vi "init_motorsystem.vi"(7 "dimension names":string[](array[string]), 8 "error in (no error)":errorcluster caption="错误输入（无错误）", 9 "CAN node IDs":u32[](array[numeric]), 10 "device index":u32, 11 "MotorSystem 输入":refnum<class "MotorSystem.lvclass">) -> (0 "error out":errorcluster caption="错误输出", 3 "MotorSystem 输出":refnum<class "MotorSystem.lvclass">)   [LabVIEW 2016, in "MotionControl.lvlib" / "MotorSystem.lvclass"]
uses:
  <userlib>/MotionControl/MotorSystem/MotorSystem.lvclass
  <userlib>/MotionControl/MotorSystem/MotorSystem.lvclass/MotorSystem.ctl
  <userlib>/MotionControl/OneMotion/OneMotion.lvclass
  <userlib>/MotionControl/MotorSystem/MotionCluster.ctl
  <vilib>/Utility/config.llb/NI_LVConfig.lvlib
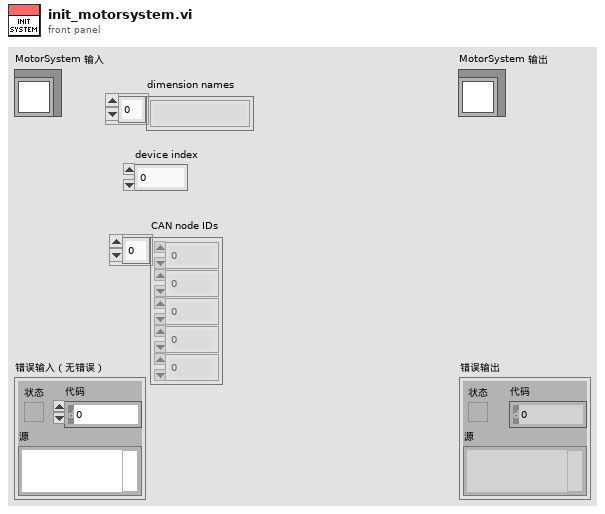
[diagram p1: front panel]
types:
  T1 = typedef "MotionControl.lvlib/MotorSystem.lvclass/MotionCluster.ctl" = cluster{"OneMotion.lvclass":refnum<class "OneMotion.lvclass">, "connected?":bool, "default enabled?":bool, "enabled?":bool}
  T2 = typedef "NI_LVConfig.lvlib/Config Data RefNum.ctl" = refnum<k1>
  T3 = typedef "MotionControl.lvlib/MotorSystem.lvclass/SavedPosCluster.ctl" = cluster{"name":string, "command list":T4}
  T4 = typedef "MotionControl.lvlib/MotorSystem.lvclass/CommandList.ctl" = cluster{"cmd":T5, "cmd info":T6[]}[]
  T5 = typedef "MotionControl.lvlib/MotorSystem.lvclass/cmd_system.ctl" = enum16{"NONE", "MOVE_SYSTEM", "WAIT_UNTIL_MOVE_DONE", "EXIT"}
  T6 = typedef "MotionControl.lvlib/MotorSystem.lvclass/SavedDimensionCluster.ctl" = cluster{"dimension name":string, "pos":dbl, "unit mode":T7, "unit conversion ratio":dbl}
  T7 = typedef "MotionControl.lvlib/OneMotion.lvclass/unit mode.ctl" = enum16{"motor (pulse)", "linear (mm) or radial (degree)"}
  T8 = cluster{"array for a soft limit":cluster{"dim name":string, "soft limit":cluster{"min":dbl, "max":dbl}}[]}[]
  T9 = cluster{"complete dimension names[0]":string, "complete dimension names[1]":string}
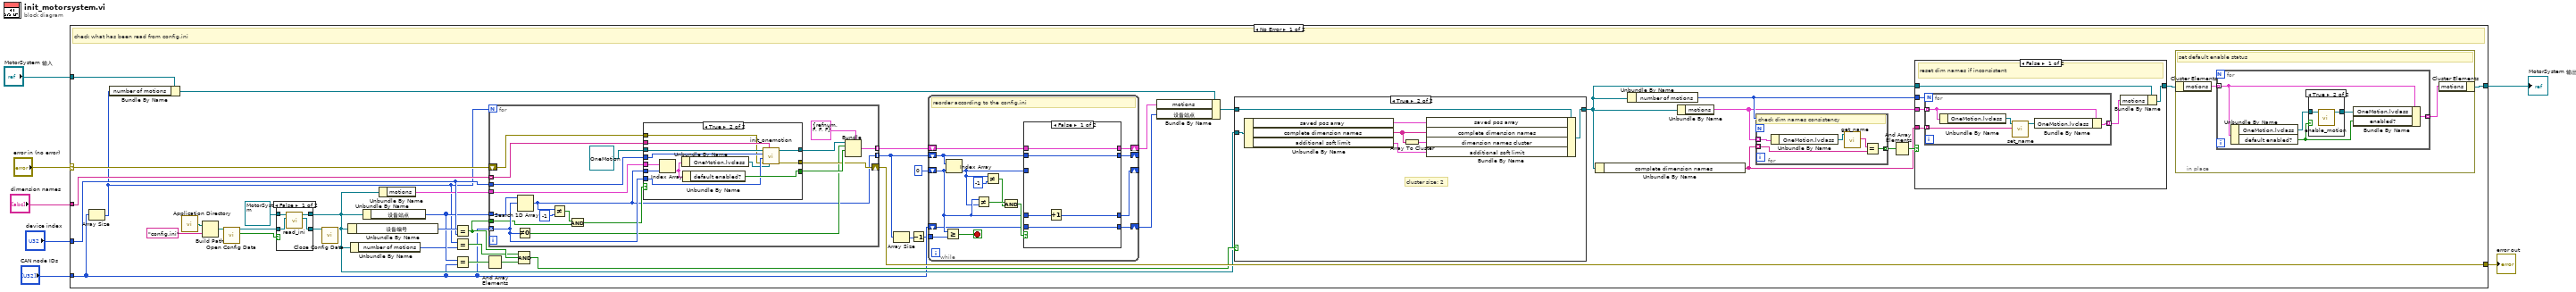
[diagram p0: block diagram]
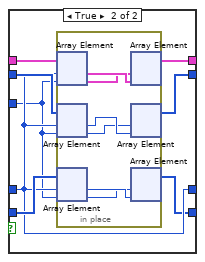
[diagram p2: hidden frame]
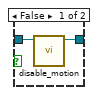
[diagram p3: hidden frame]
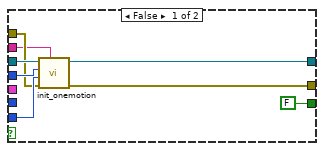
[diagram p7: hidden frame]
diagram:
  n1 = case shown="No Error" "error in (no error)" {
    selector: "error in (no error)" -> [w47 w164]
    tunnel: [w45 w164] -> w6
    tunnel: [w16 w163] -> w4
    tunnel: "MotorSystem 输入" -> [w46 w163]
    tunnel: "CAN node IDs" -> [w11 _]
    tunnel: "device index" -> [w36 _]
    tunnel: "dimension names" -> [w44 _]
    frame No Error {
      # "check what has been read from config.ini"
      n2 = Array Size(array=w11) -> (size(s)=w32:i32)
      n3 = Bundle By Name(cluster=w46, "number of motions"=w32) -> (w48:refnum<class "MotorSystem.lvclass">)
      n4 = call <vilib>:"Application Directory.vi"() -> ("Application Directory"=w43:path)
      n5 = Build Path(base path=w43, name or relative path="config.ini" ("名称或相对路径")) -> (appended path=w38:path)
      n6 = call <vilib>:"Open Config Data.vi"("configuration file path"=w38) -> ("file created?"=w18:bool, "refnum"=w41:T2)  [unwired: 8 in, 1 out]
      n7 = case shown="False" w18 {
        tunnel: w41 -> [w97 w98]
        tunnel: [w96 w98] -> w40
        tunnel: refnum<class "MotorSystem.lvclass"> refnum ("MotorSystem.lvclass") -> [w95 w99]
        tunnel: [w94 w99] -> w26
        frame False {
          n8 = call-dynamic "read_ini.vi"("file ref in"=w97, "MotorSystem 输入"=w95) -> ("file ref out"=w96:T2, "MotorSystem 输出"=w94:refnum<class "MotorSystem.lvclass">)  [unwired: 7 in, 1 out]
        }
        frame True {
        }
      }
      n9 = call <vilib>:"Close Config Data.vi"("refnum"=w40) -> ()  [unwired: 9 in, 2 out]
      n10 = Unbundle By Name(w26) -> ("设备编号"=w37:u32)
      n11 = Unbundle By Name(w26) -> ("number of motions"=w31:i32)
      n12 = Unbundle By Name(w26) -> ("设备站点"=w34:u32[])
      n13 = Unbundle By Name(w26) -> ("motions"=w35:T1[])
      n14 = Equal?(x=w37, y=w36) -> (x = y?=w30:bool)
      n15 = Equal?(x=w32, y=w31) -> (x = y?=w29:bool)
      n16 = Equal?(x=w34, y=w11) -> (x = y?=w33:bool[])
      n17 = And Array Elements(Boolean array=w33) -> (logical AND=w28:bool)
      n18 = for {
        N: w32 -> [_]
        tunnel: w11 -> [w130] mode=indexing
        tunnel: [w141] -> w15 mode=indexing
        shift-right: [w131] -> w45
        shift-left: w47 -> [w132]
        tunnel: w36 -> [w133]
        tunnel: w44 -> [w134] mode=indexing
        tunnel: w30 -> [w127]
        tunnel: w34 -> [w140]
        tunnel: w35 -> [w138]
        tunnel: [w125] -> w12 mode=indexing
        n19 = Not Equal To 0?(x=w130) -> (x != 0?=w129:bool)
        n20 = Search 1D Array(1D array=w140, element=w130) -> (index of element=w125:i32)  [unwired: 1 in]
        n21 = Not Equal?(x=w125, y=-1) -> (x != y?=w126:bool)
        n22 = And(x=w126, y=w127) -> (x .and. y?=w128:bool)
        n23 = case shown="True" w128 {
          tunnel: w138 -> [_ w162]
          tunnel: w125 -> [_ w161]
          tunnel: [w148 w152] -> w137
          tunnel: [FALSE ("enabled?") w159] -> w136
          tunnel: refnum<class "OneMotion.lvclass"> refnum ("OneMotion.lvclass") -> [w149 w158]
          tunnel: w134 -> [w143 w157]
          tunnel: w133 -> [w146 w156]
          tunnel: w130 -> [w147 w155]
          tunnel: w132 -> [w145 w154]
          tunnel: [w144 w153] -> w131
          frame False {
            n24 = call <userlib>:"init_onemotion.vi"("dimension name"=w143, "error in (no error)"=w145, "CAN node ID"=w147, "device index"=w146, "OneMotion 输入"=w149) -> ("error out"=w144:errorcluster, "OneMotion 输出"=w148:refnum<class "OneMotion.lvclass">)  [unwired: 5 in]
          }
          frame True {
            n25 = Index Array(array=w162, index=w161) -> (element=w160:T1)
            n26 = Unbundle By Name(w160) -> ("OneMotion.lvclass"=w151:refnum<class "OneMotion.lvclass">)
            n27 = Unbundle By Name(w160) -> ("default enabled?"=w159:bool)
            n28 = call <userlib>:"init_onemotion.vi"("OneMotion from file"=w151, "dimension name"=w157, "error in (no error)"=w154, "CAN node ID"=w155, "device index"=w156, "OneMotion 输入"=w158) -> ("error out"=w153:errorcluster, "OneMotion 输出"=w152:refnum<class "OneMotion.lvclass">)  [unwired: 4 in]
          }
        }
        n29 = Bundle(cluster=T1 {"OneMotion.lvclass"=refnum, "connected?"=FALSE, "default enabled?"=FALSE, "enabled?"=FALSE} ("簇"), "OneMotion.lvclass"=w137, "connected?"=w129, "default enabled?"=w136) -> (w141:T1)  [unwired: 1 in]
      }
      n30 = Compound Arithmetic op=AND(w29, w30, w28) -> (w27:bool)
      n31 = Array Size(array=w12) -> (size(s)=w13:i32)
      n32 = Decrement(x=w13) -> (x-1=w8:i32)
      n33 = while {
        shift-right: [w57] -> _
        shift-left: 0 -> [w54]
        shift-right: [w59] -> w14
        shift-left: w15 -> [w60]
        tunnel: w8 -> [w56]
        shift-right: [w51] -> _
        shift-left: w12 -> [w52]
        shift-right: [w49] -> w10
        shift-left: w11 -> [w50]
        stop <- w55 stop-if-true
        # "reorder according to the config.ini"
        n34 = Greater Or Equal?(x=w54, y=w56) -> (x >= y?=w55:bool)
        n35 = Index Array(array=w52, index=w54) -> (element=w53:i32)
        n36 = Not Equal?(x=w54, y=w53) -> (x != y?=w62:bool)
        n37 = Not Equal?(x=w53, y=-1) -> (x != y?=w61:bool)
        n38 = And(x=w62, y=w61) -> (x .and. y?=w58:bool)
        n39 = case shown="False" w58 {
          tunnel: w60 -> [w68 w76]
          tunnel: w54 -> [w67 w71]
          tunnel: w53 -> [_ w70]
          tunnel: [w68 w75] -> w59
          tunnel: [w66 w71] -> w57
          tunnel: w52 -> [w65 w74]
          tunnel: [w65 w73] -> w51
          tunnel: w50 -> [w64 w72]
          tunnel: [w64 w69] -> w49
          frame False {
            n40 = Increment(x=w67) -> (x+1=w66:i32)
          }
          frame True {
            n41 = in-place {
              n42 = in-place-array #1(w76, w71, w70) -> (w82:T1, w81:T1)
              n43 = in-place-array #2(w74, w71, w70) -> (w80:i32, w79:i32)
              n44 = in-place-array #3(w72, w71, w70) -> (w78:u32, w77:u32)
              n45 = in-place-array #1(w81, w82) -> (w75:T1[])  [unwired: 2 out]
              n46 = in-place-array #2(w79, w80) -> (w73:i32[])  [unwired: 2 out]
              n47 = in-place-array #3(w77, w78) -> (w69:u32[])  [unwired: 2 out]
            }
          }
        }
      }
      n48 = Bundle By Name(cluster=w48, "motions"=w14, "设备站点"=w10) -> (w25:refnum<class "MotorSystem.lvclass">)
      n49 = case shown="True" w27 {
        tunnel: w26 -> [_ w122]
        tunnel: w25 -> [w117 w124]
        tunnel: [w117 w119] -> w19
        frame False {
        }
        frame True {
          # "cluster size: 2"
          n50 = Unbundle By Name(w122) -> ("saved pos array"=w123:T3[], "complete dimension names"=w121:string[], "additional soft limit"=w118:T8)
          n51 = Array To Cluster(array=w121) -> (cluster=w120:T9)
          n52 = Bundle By Name(cluster=w124, "saved pos array"=w123, "complete dimension names"=w121, "dimension names cluster"=w120, "additional soft limit"=w118) -> (w119:refnum<class "MotorSystem.lvclass">)
        }
      }
      n53 = Unbundle By Name(w19) -> ("complete dimension names"=w20:string[])
      n54 = Unbundle By Name(w19) -> ("number of motions"=w22:i32)
      n55 = Unbundle By Name(w19) -> ("motions"=w21:T1[])
      n56 = for {
        N: w22 -> [_]
        tunnel: w21 -> [w116] mode=indexing
        tunnel: w20 -> [w113] mode=indexing
        tunnel: [w112] -> w24 mode=indexing
        # "check dim names consistency"
        n57 = Unbundle By Name(w116) -> ("OneMotion.lvclass"=w115:refnum<class "OneMotion.lvclass">)
        n58 = call-dynamic "get_name.vi"("OneMotion输入"=w115) -> ("name"=w114:string)  [unwired: 8 in, 2 out]
        n59 = Equal?(x=w114, y=w113) -> (x = y?=w112:bool)
      }
      n60 = And Array Elements(Boolean array=w24) -> (logical AND=w23:bool)
      n61 = case shown="False" w23 {
        tunnel: w22 -> [w105 _]
        tunnel: w21 -> [w104 _]
        tunnel: w20 -> [w103 _]
        tunnel: w19 -> [w102 w111]
        tunnel: [w100 w111] -> w17
        frame False {
          # "reset dim names if inconsistent"
          n62 = for {
            N: w105 -> [_]
            tunnel: w104 -> [w108] mode=indexing
            tunnel: w103 -> [w109] mode=indexing
            tunnel: [w106] -> w101 mode=indexing
            n63 = Unbundle By Name(w108) -> ("OneMotion.lvclass"=w110:refnum<class "OneMotion.lvclass">)
            n64 = call-dynamic "set_name.vi"("name"=w109, "OneMotion输入"=w110) -> ("OneMotion输出"=w107:refnum<class "OneMotion.lvclass">)  [unwired: 8 in, 1 out]
            n65 = Bundle By Name(cluster=w108, "OneMotion.lvclass"=w107) -> (w106:T1)
          }
          n66 = Bundle By Name(cluster=w102, "motions"=w101) -> (w100:refnum<class "MotorSystem.lvclass">)
        }
        frame True {
        }
      }
      n67 = in-place {
        # "set default enable status"
        n68 = in-place-cluster #4(w17) -> ("motions"=w84:T1[])
        n69 = for {
          tunnel: w84 -> [w88] mode=indexing
          tunnel: [w85] -> w83 mode=indexing
          n70 = Unbundle By Name(w88) -> ("OneMotion.lvclass"=w89:refnum<class "OneMotion.lvclass">, "default enabled?"=w86:bool)
          n71 = case shown="True" w86 {
            tunnel: w89 -> [w91 w93]
            tunnel: [w90 w92] -> w87
            frame False {
              n72 = call <userlib>:"disable_motion.vi"("OneMotion 输入"=w91) -> ("OneMotion 输出"=w90:refnum<class "OneMotion.lvclass">)  [unwired: 9 in, 1 out]
            }
            frame True {
              n73 = call <userlib>:"enable_motion.vi"("OneMotion 输入"=w93) -> ("OneMotion 输出"=w92:refnum<class "OneMotion.lvclass">)  [unwired: 9 in, 1 out]
            }
          }
          n74 = Bundle By Name(cluster=w88, "OneMotion.lvclass"=w87, "enabled?"=w86) -> (w85:T1)
        }
        n75 = in-place-cluster #4("motions"=w83) -> (w16:refnum<class "MotorSystem.lvclass">)
      }
    }
    frame Error {
    }
  }
  "error out" <- w6
  "MotorSystem 输出" <- w4
